vi "Bits to Bytes.vi"(11 "Bits":bool[](array[boolean])) -> (2 "Bytes":u8[](array[numeric]), 3 "Count":u8)   [LabVIEW 2021]
doc: "Converts an array of bits into an array of bytes."
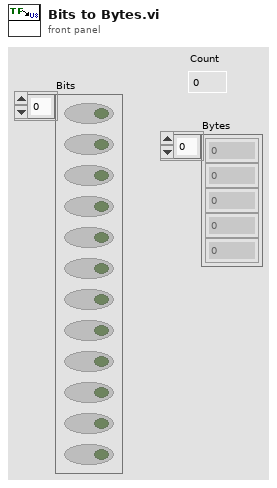
[diagram p1: front panel]
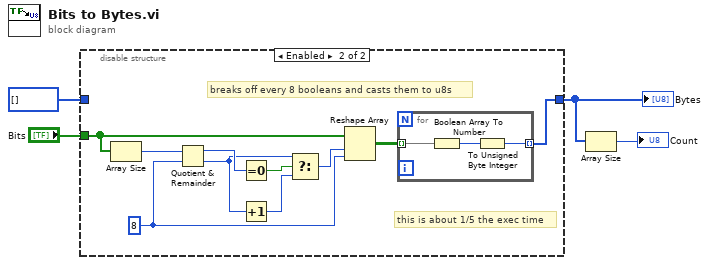
[diagram p0: block diagram]
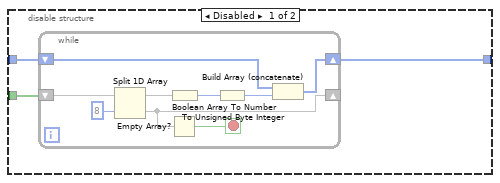
[diagram p2: hidden frame]
diagram:
  n1 = disable-structure shown="Enabled" {
    disable-tunnel: u8[] [] ("data Return") -> [w7 _]
    disable-tunnel: "Bits" -> [w6 w21]
    disable-tunnel: [w5 w17] -> w2
    frame Disabled {
      n2 = while {
        shift-right: [w12] -> _
        shift-left: w6 -> [w16]
        shift-right: [w13] -> w5
        shift-left: w7 -> [w14]
        stop <- w11 stop-if-true
        n3 = Split 1D Array(array=w16, index=8) -> (first subarray=w10:bool[], second subarray=w12:bool[])
        n4 = Empty Array?(array=w12) -> (empty?=w11:bool)
        n5 = Boolean Array To Number(Boolean array=w10) -> (number=w9:u32)
        n6 = To Unsigned Byte Integer(number=w9) -> (unsigned 8bit integer=w8:u8)
        n7 = Build Array (concatenate)(w14, w8) -> (w13:u8[])
      }
    }
    frame Enabled {
      w19 = 8 ("y")
      # "this is about 1/5 the exec time"
      # "breaks off every 8 booleans and casts them to u8s"
      n8 = Array Size(array=w21) -> (size(s)=w26:i32)
      n9 = Quotient & Remainder(x=w26, y=w19) -> (x-y*floor(x/y)=w25:i32, floor(x/y)=w22:i32)
      n10 = Equal To 0?(x=w25) -> (x = 0?=w24:bool)
      n11 = Increment(x=w22) -> (x+1=w23:i32)
      n12 = Select(t=w22, s=w24, f=w23) -> (s? t:f=w20:i32)
      n13 = Reshape Array(w21, w20, w19) -> (w18:bool[][])
      n14 = for {
        tunnel: w18 -> [w28] mode=indexing
        tunnel: [w29] -> w17 mode=indexing
        n15 = Boolean Array To Number(Boolean array=w28) -> (number=w27:u32)
        n16 = To Unsigned Byte Integer(number=w27) -> (unsigned 8bit integer=w29:u8)
      }
    }
  }
  "Bytes" <- w2
  n17 = Array Size(array=w2) -> (size(s)=→"Count":i32)
